vi "Run Action_Do.vi"(8 "error in (no error)":errorcluster, 10 "Project Builder in":refnum<class "Project Builder.lvclass">, 11 "Report":refnum<class "Report Action.lvclass">) -> (0 "error out":errorcluster, 1 "Success?":bool, 3 "Report":refnum<class "Report Data.lvclass">)   [LabVIEW 2019, in "ProjectBuilder.lvlib" / "Report Action.lvclass"]
doc: "This implementation does nothing but return 'Success?'=False as the method is not inteded to ever be called."
uses:
  Report Action.lvclass
  Data/Report Data/Report Data.lvclass
  Project Builder/Project Builder.lvclass
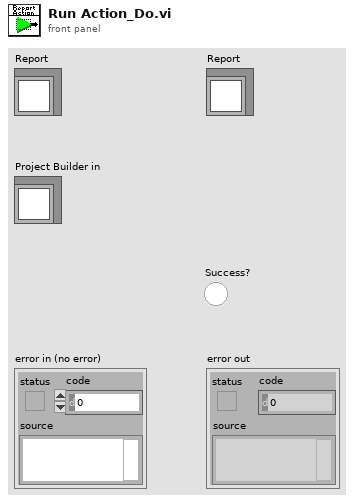
[diagram p1: front panel]
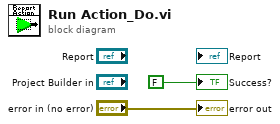
[diagram p0: block diagram]
diagram:
  "error out" <- "error in (no error)"
  "Success?" <- FALSE
